vi "SET_DAC.vi"(2 "error in (no error)":errorcluster, 3 "Input":i32(knob)=3000 min=-5000 max=5000 scale=-5000.0..5000.0, 4 "VISA resource Input":refnum<visa-resource-name>) -> (0 "error out":errorcluster, 1 "VISA resource Quit":refnum<visa-resource-name>)   [LabVIEW 2011]
panel:
  out "unsigned byte array":u8[](array[numeric])
  out "Input 2":i32=127
  out "Read SET_DAC command":u8[](array[numeric])
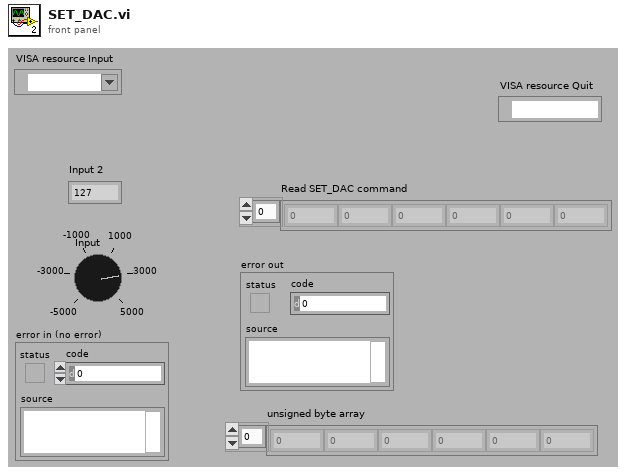
[diagram p1: front panel]
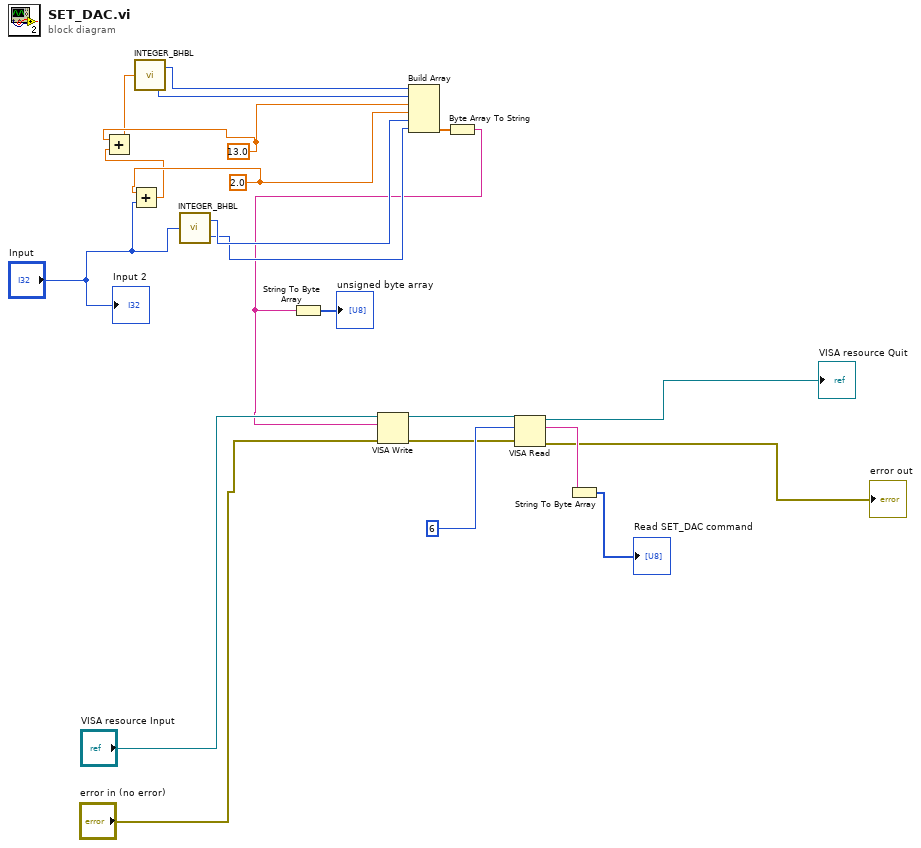
[diagram p0: block diagram]
diagram:
  w8 = 2.0 ("element")
  w6 = 13.0 ("element")
  n1 = Add(x=w8, y="Input") -> (x+y=w7:dbl)
  n2 = Add(x=w6, y=w7) -> (x+y=w5:dbl)
  n3 = call "INTEGER_BHBL.vi"("int16"=w5) -> ("Lvalue"=w3:u8, "HValue"=w4:u8)
  n4 = call "INTEGER_BHBL.vi"("int16"="Input") -> ("Lvalue"=w10:u8, "HValue"=w11:u8)
  n5 = Build Array(w4, w3, w6, w8, w11, w10) -> (w14:dbl[])
  n6 = Byte Array To String(unsigned byte array=w14) -> (string=w2:string)
  n7 = String To Byte Array(string=w2) -> (unsigned byte array=→"unsigned byte array":u8[])
  n8 = VISA Write(VISA resource name="VISA resource Input", write buffer=w2, error in (no error)="error in (no error)") -> (VISA resource name out=w15:refnum<visa-resource-name>, error out=w17:errorcluster)  [unwired: 1 out]
  n9 = VISA Read(VISA resource name=w15, byte count=u32 6, error in (no error)=w17) -> (VISA resource name out=→"VISA resource Quit":refnum<visa-resource-name>, read buffer=w20:string, error out=→"error out":errorcluster)  [unwired: 1 out]
  n10 = String To Byte Array(string=w20) -> (unsigned byte array=→"Read SET_DAC command":u8[])
  "Input 2" <- "Input"
